vi "add_elementToHostMessages_p.vi"(0 "MoAgSy_Host":refnum<class "MoAgSy_Host.lvclass">, 3 "MoAgSy_Message":refnum<class "MoAgSy_Message.lvclass">, 5 "error in (no error)":errorcluster) -> (14 "dup MoAgSy_Host":refnum<class "MoAgSy_Host.lvclass">, 19 "error out":errorcluster)   [LabVIEW 2009, in "MoAgSy.lvlib" / "MoAgSy_Host.lvclass"]
doc: "<B>protected</B> VI adds new incoming host messages to hosts message array.\nThis array contains all new host messages and is flushed in the host message handler section of a run host vi\n\nF.Berck@gsi.de\nGSI Darmstadt 2009"
uses:
  MoAgSy_Host.lvclass
  MoAgSy_Message/MoAgSy_Message.lvclass
  MoAgSy_Host.lvclass/MoAgSy_Host.ctl
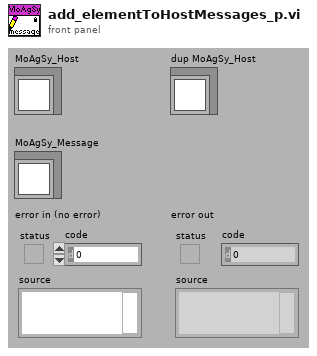
[diagram p1: front panel]
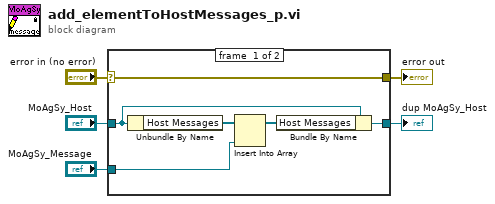
[diagram p0: block diagram]
diagram:
  n1 = case shown="No Error" "error in (no error)" {
    selector: "error in (no error)" -> [w11 w12]
    tunnel: [w11 w12] -> w4
    tunnel: [w10 w13] -> w2
    tunnel: "MoAgSy_Host" -> [w9 w13]
    tunnel: "MoAgSy_Message" -> [w6 _]
    frame #0 {
      n2 = Unbundle By Name(w9) -> ("Host Messages"=w8:refnum<class "MoAgSy_Message.lvclass">[])
      n3 = Insert Into Array(array=w8, new element=w6) -> (w7:refnum<class "MoAgSy_Message.lvclass">[])  [unwired: 1 in]
      n4 = Bundle By Name(cluster=w9, "Host Messages"=w7) -> (w10:refnum<class "MoAgSy_Host.lvclass">)
    }
    frame #1 {
    }
  }
  "error out" <- w4
  "dup MoAgSy_Host" <- w2
